vi "Create.vi"(7 "Shared Resource (F)":bool, 8 "error in (no error)":errorcluster, 10 "Subsystem Name (optional)":string, 11 "SMO":refnum<class "SMO.lvclass">) -> (0 "error out":errorcluster, 2 "SMO name":string, 3 "SMO out":refnum<class "SMO.lvclass">)   [LabVIEW 2019, in "SMO.lvclass"]
doc: "Constructor\n\n\n---------------------------------------------------------------\nJKI State Machine Objects™\nhttp://jki.net/state-machine-objects/\nCopyright (C) 2005-2015, JKI <info@jki.net>\nALL RIGHTS RESERVEDJKI State Machine Objects (SMO) 1.3.0.56\nJKI - JKI\nCopyright (c) 2017, JKI"
uses:
  SMO.lvclass
  SMO.lvclass/SMO.ctl
  Typedefs/Process Error Notification--Cluster.ctl
  Typedefs/SMOState --Enum.ctl
  Support/Attribute.Identity/Attribute.Identity.lvclass
  C:/Users/Patrick/Documents/GitHub/Test (LV2019)/lv-venv/lv.lib/vi.lib/JKI/JKI SMO/Support/Attribute/Attribute.lvclass
  Registry/Registry-SMO.lvclass
panel:
  # "For instructions on how to use the JKI State Machine Objects, examples and video tutorials, visit:\nhttp://jki.net/state-machine-objects/\n\nJKI State Machine Objects™\nhttp://jki.net/state-machine-objects/\nCopyright (C) 2005-2015, JKI <info@jki.net>\nALL RIGHTS RESERVED"
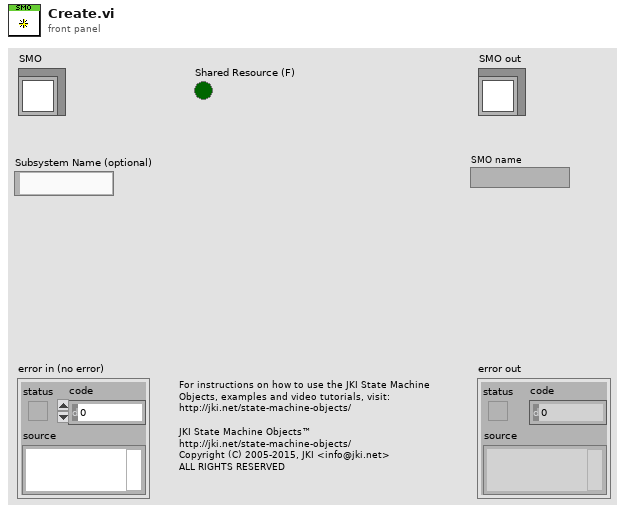
[diagram p1: front panel]
types:
  T1 = typedef "SMO.lvclass/SMOState --Enum.ctl" = enum16{"unknown", "Created", "Started", "Stopped"}
  T2 = typedef "SMO.lvclass/Process Error Notification--Cluster.ctl" = cluster{"error":errorcluster}
  T3 = typedef "SMO.lvclass/PrivateData--Ref.ctl" = refnum<data-value>
  T4 = typedef "SMO.lvclass/PrivateData--Cluster.ctl" = cluster{"Parent Call":T5, "Registered Processes":T6[], "Sync Notifier":refnum<notifier>, "Process Error Notifier":refnum<notifier>, "Protected Events":T7, "Public Events":T8, "SMO State":T1, "[Dependencies]":T9[], "[Attributes]":refnum<class "Attribute.lvclass">[], "Launcher Close":refnum<notifier>, "Caller Watchdog":refnum<queue>, "Accessibility":T10, "NbStaticDependencies":u32}
  T5 = typedef "SMO.lvclass/Parent Call--Enum.ctl" = enum16{"Allows parent to run", "Does not request parent to run"}
  T6 = typedef "SMO.lvclass/RegisteredProcessData--Cluster.ctl" = cluster{"Name":string, "Static VI Ref":refnum<vi>, "Running":bool, "NotifierRef":u32}
  T7 = typedef "SMO.lvclass/Protected Events.ctl" = cluster{"StopProcesses":refnum<user-event>, "AbortProcesses":refnum<user-event>, "Config Changed":refnum<user-event>, "Dependency":refnum<user-event>}
  T8 = typedef "SMO.lvclass/Public Events.ctl" = cluster{"Error":refnum<user-event>, "State":refnum<user-event>, "Reserve State":refnum<user-event>}
  T9 = typedef "SMO.lvclass/SMO Dependency--Cluster.ctl" = cluster{"Dependency":refnum<class "SMO.lvclass">, "Level":string}
  T10 = typedef "SMO.lvclass/Accessibility--Cluster.ctl" = cluster{"Lock Key":string, "Reserve State":T11}
  T11 = typedef "SMO.lvclass/Reserve State--Enum.ctl" = enum16{"Unreserved", "Reserved", "Self-locked"}
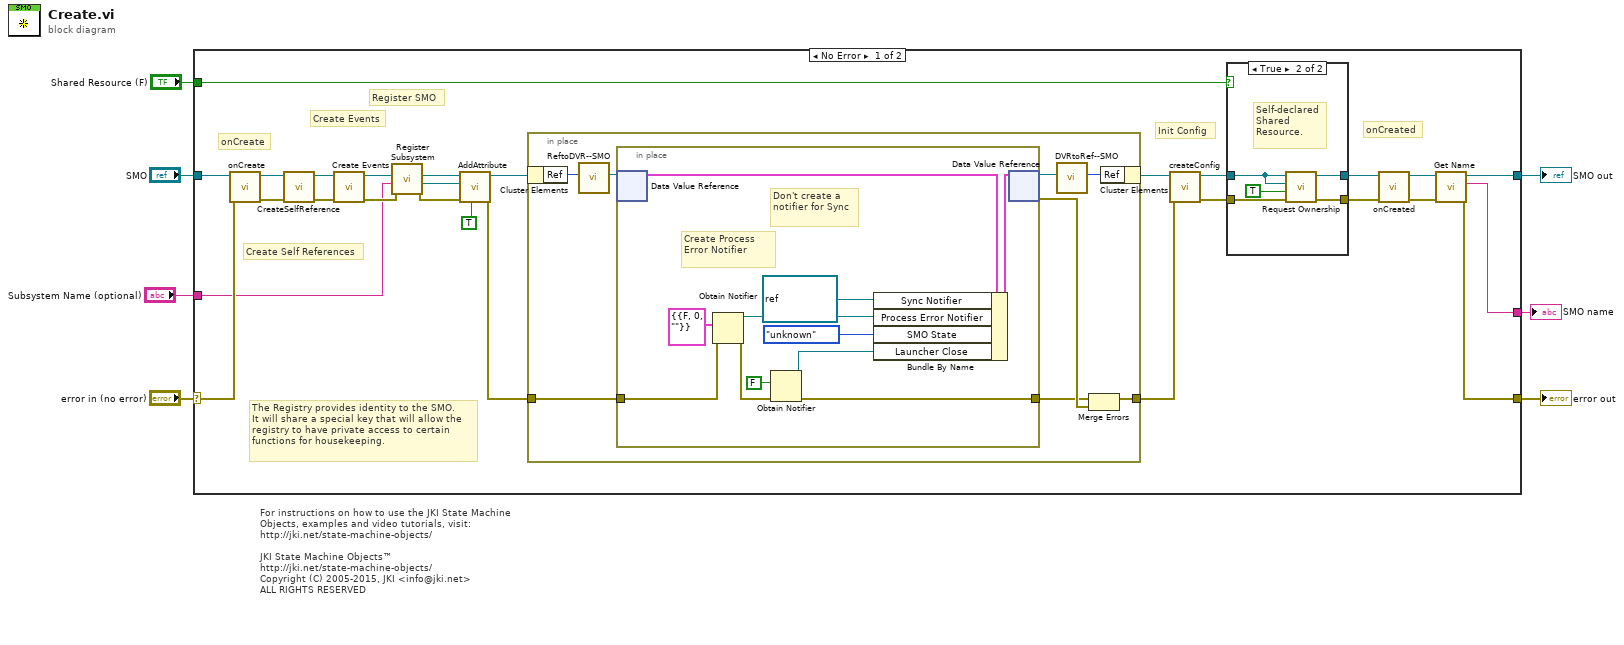
[diagram p0: block diagram]
diagram:
  # "For instructions on how to use the JKI State Machine Objects, examples and video tutorials, visit:\nhttp://jki.net/state-machine-objects/\n\nJKI State Machine Objects™\nhttp://jki.net/state-machine-objects/\nCopyright (C) 2005-2015, JKI <info@jki.net>\nALL RIGHTS RESERVED"
  n1 = case shown="No Error" "error in (no error)" {
    selector: "error in (no error)" -> [w31 w62]
    tunnel: [w26 w62] -> w6
    tunnel: [w28 w61] -> w4
    tunnel: "SMO" -> [w32 w61]
    tunnel: "Subsystem Name (optional)" -> [w30 _]
    tunnel: [w25 _] -> w2
    tunnel: "Shared Resource (F)" -> [w8 _]
    frame No Error {
      # "Init Config"
      # "The Registry provides identity to the SMO.\nIt will share a special key that will allow the\nregistry to have private access to certain\nfunctions for housekeeping."
      # "Create Self References"
      # "onCreated"
      # "Register SMO"
      # "Create Events"
      # "onCreate"
      n2 = call-dynamic "onCreate.vi"("error in (no error)"=w31, "SMO"=w32) -> ("error out"=w18:errorcluster, "SMO out"=w20:refnum<class "SMO.lvclass">)  [unwired: 8 in]
      n3 = call-dynamic "CreateSelfReference.vi"("error in (no error)"=w18, "SMO"=w20) -> ("error out"=w17:errorcluster, "SMO out"=w19:refnum<class "SMO.lvclass">)  [unwired: 8 in]
      n4 = call "Create Events.vi"("error in (no error)"=w17, "SMO"=w19) -> ("error out"=w33:errorcluster, "SMO out"=w34:refnum<class "SMO.lvclass">)  [unwired: 8 in]
      n5 = call "Register Subsystem.vi"("error in (no error)"=w33, "Subsystem Name (optional)"=w30, "JKI SMO in"=w34) -> ("error out"=w22:errorcluster, "Attribute.Identity"=w16:refnum<class "Attribute.Identity.lvclass">, "JKI SMO out"=w24:refnum<class "SMO.lvclass">)  [unwired: 6 in]
      n6 = call "AddAttribute.vi"("Overwrite? (F)"=TRUE, "error in (no error)"=w22, "Attribute"=w16, "SMO in"=w24) -> ("error out"=w21:errorcluster, "SMO out"=w23:refnum<class "SMO.lvclass">)  [unwired: 6 in]
      n7 = in-place {
        in-place-border: [w48] -> w13
        in-place-border: w21 -> [w46]
        n8 = in-place-cluster #1(w23) -> ("Ref"=w45:u32)
        n9 = call "ReftoDVR--SMO.vi"("Ref"=w45) -> ("Ref"=w44:T3)  [unwired: 10 in]
        n10 = in-place {
          in-place-border: [w51] -> w47
          in-place-border: w46 -> [w56]
          # "Don't create a notifier for Sync"
          # "Create Process Error Notifier"
          n11 = in-place-dvr #2(w44) -> (w60:T4)  [unwired: 1 out]
          n12 = Obtain Notifier(notification data type=T2 {"error"={"status"=FALSE, "code"=0, "source"=""}} ("Process Notification"), error in (no error)=w56) -> (notifier out=w58:refnum<notifier>, error out=w52:errorcluster)  [unwired: 2 in, 1 out]
          n13 = Obtain Notifier(notification data type=FALSE ("Launcher Close"), error in (no error)=w52) -> (notifier out=w50:refnum<notifier>, error out=w51:errorcluster)  [unwired: 2 in, 1 out]
          n14 = Bundle By Name(cluster=w60, "Sync Notifier"=refnum<notifier> refnum, "Process Error Notifier"=w58, "SMO State"=SMOState_--Enum."unknown", "Launcher Close"=w50) -> (w59:T4)
          n15 = in-place-dvr #2(w59) -> (w43:T3, w49:errorcluster)
        }
        n16 = call "DVRtoRef--SMO.vi"("Ref"=w43) -> ("Ref"=w42:u32)  [unwired: 10 in]
        n17 = Merge Errors(w47, w49) -> (w48:errorcluster)
        n18 = in-place-cluster #1("Ref"=w42) -> (w14:refnum<class "SMO.lvclass">)
      }
      n19 = call "createConfig.vi"("error in (no error)"=w13, "SMO in"=w14) -> ("error out"=w11:errorcluster, "SMO out"=w9:refnum<class "SMO.lvclass">)  [unwired: 8 in]
      n20 = case shown="True" w8 {
        tunnel: [w36 w41] -> w12
        tunnel: w11 -> [w35 w40]
        tunnel: [w35 w39] -> w10
        tunnel: w9 -> [w36 w38]
        frame False {
        }
        frame True {
          # "Self-declared\nShared\nResource."
          n21 = call "Request Ownership.vi"("error in (no error)"=w40, "Shared Resource"=TRUE, "Dependency"=w38, "SMO in"=w38) -> ("error out"=w39:errorcluster, "SMO out"=w41:refnum<class "SMO.lvclass">)  [unwired: 5 in, 1 out]
        }
      }
      n22 = call-dynamic "onCreated.vi"("error in (no error)"=w10, "SMO"=w12) -> ("error out"=w27:errorcluster, "SMO out"=w29:refnum<class "SMO.lvclass">)  [unwired: 8 in]
      n23 = call "Get Name.vi"("error in (no error)"=w27, "SMO"=w29) -> ("error out"=w26:errorcluster, "Name"=w25:string, "SMO out"=w28:refnum<class "SMO.lvclass">)  [unwired: 7 in]
    }
    frame Error {
    }
  }
  "error out" <- w6
  "SMO out" <- w4
  "SMO name" <- w2
